vi "getKey.vi"(7 "payload":u8[](array[numeric]), 11 "Rx":u8[](array[numeric])=[2, 39, 2]) -> (3 "Keyload":u8[](array[numeric]))   [LabVIEW 2018]
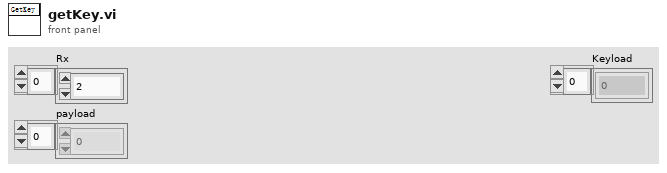
[diagram p1: front panel]
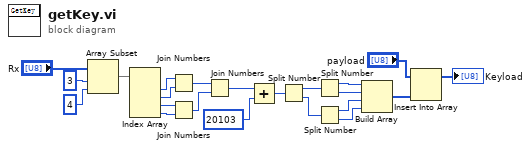
[diagram p0: block diagram]
diagram:
  n1 = Array Subset(array="Rx", index=3, length=4) -> (w5:u8[])
  n2 = Index Array(array=w5) -> (element #1=w7:u8, element #2=w8:u8, element #3=w9:u8, element #4=w10:u8)  [unwired: 4 in]
  n3 = Join Numbers(hi=w7, lo=w8) -> ((hi.lo)=w11:u16)
  n4 = Join Numbers(hi=w9, lo=w10) -> ((hi.lo)=w12:u16)
  n5 = Join Numbers(hi=w11, lo=w12) -> ((hi.lo)=w13:u32)
  n6 = Add(x=w13, y=u32 20103) -> (x+y=w14:u32)
  n7 = Split Number(x=w14) -> (hi(x)=w15:u16, lo(x)=w16:u16)
  n8 = Split Number(x=w15) -> (hi(x)=w17:u8, lo(x)=w18:u8)
  n9 = Split Number(x=w16) -> (hi(x)=w19:u8, lo(x)=w20:u8)
  n10 = Build Array(w17, w18, w19, w20) -> (w4:u8[])
  n11 = Insert Into Array(array="payload", new element=w4) -> (→"Keyload":u8[])  [unwired: 1 in]
